vi "Split Error Cluster Array.vi"(0 "Error cluster array":errorcluster[](array[cluster])) -> (1 "status":bool[](array[boolean]), 2 "codes":i32[](array[numeric]), 3 "msg":string[](array[string]))   [LabVIEW 2020]
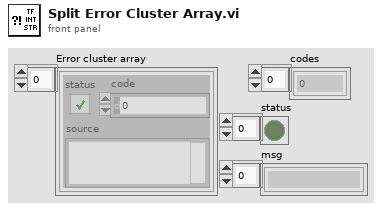
[diagram p1: front panel]
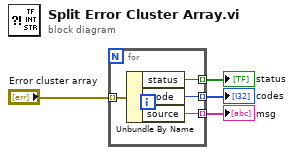
[diagram p0: block diagram]
diagram:
  n1 = for {
    tunnel: "Error cluster array" -> [w8] mode=indexing
    tunnel: [w7] -> w2 mode=indexing
    tunnel: [w6] -> w3 mode=indexing
    tunnel: [w5] -> w1 mode=indexing
    n2 = Unbundle By Name(w8) -> ("status"=w7:bool, "code"=w6:i32, "source"=w5:string)
  }
  "codes" <- w3
  "status" <- w2
  "msg" <- w1
